vi "Create HTML.vi"(7 "FP Reference":refnum<class "Web Front Panel.lvclass">, 8 "error in (no error)":errorcluster, 10 "VI Identifier":string, 11 "Select In":refnum<class "Select.lvclass">) -> (0 "error out":errorcluster, 1 "js code for controls":string, 2 "js variables":string, 3 "Select Out":refnum<class "Select.lvclass">, 4 "script dependencies":string[](array[string]), 5 "HTML":string, 6 "js code for indicators":string)   [LabVIEW 2017, in "Front Panel Publisher.lvlib" / "Select.lvclass"]
uses:
  Select.lvclass
  Object_class/Object.lvclass
  Control_class/Control.lvclass
  Front Panel Publisher.lvlib
  Web Front Panel_class/Web Front Panel.lvclass
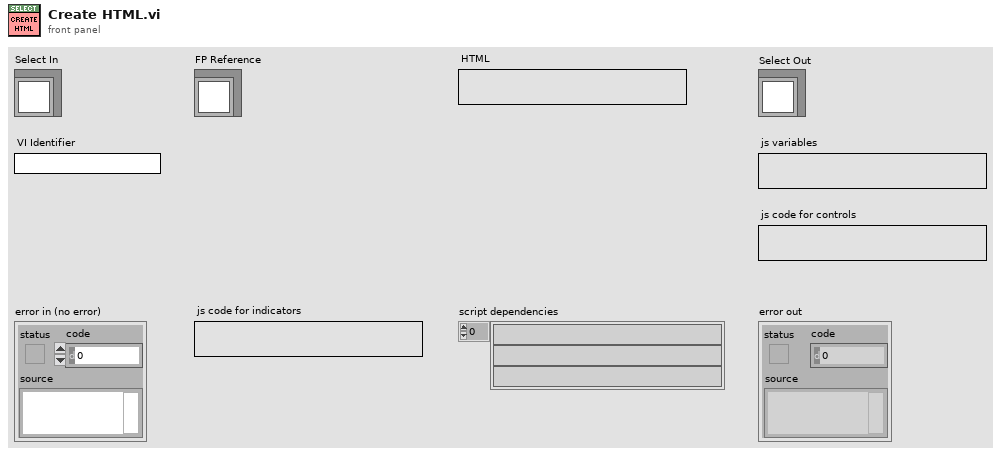
[diagram p1: front panel]
types:
  T1 = typedef "Front Panel Publisher.lvlib/Object.lvclass/Attributes.ctl" = cluster{"UID":i32, "Type":string, "Starting Location":T2, "Reference":refnum<vi>, "Cluster Component":bool, "Starting Rect Position":cluster{"Left":i16, "Top":i16}, "Owning Pane":refnum<vi>, "Master Total Rect Delta":T3}
  T2 = typedef "Front Panel Publisher.lvlib/Object.lvclass/Coordinates.ctl" = cluster{"Left":i32, "Top":i32, "Height":u32, "Width":u32}
  T3 = typedef "LVRectTypeDef.ctl" = cluster{"Left":i16, "Top":i16, "Right":i16, "Bottom":i16}
  T4 = typedef "Front Panel Publisher.lvlib/Control.lvclass/Attributes.ctl" = cluster{"Description":string, "Indicator":bool, "Default Value":variant, "Control Index":i32, "Label":refnum<class "Text.lvclass">, "Caption":refnum<class "Text.lvclass">, "Image b64":string, "No Control Index":bool, "Display Mode":T5}
  T5 = typedef "Front Panel Publisher.lvlib/Web Front Panel.lvclass/Enum - Control Display Mode.ctl" = enum16{"Value Only", "Value and Visibility", "Boolean Value Only", "Boolean Value and Visibility", "Control is Image", "Image and Visibility"}
  T6 = typedef "Front Panel Publisher.lvlib/Select.lvclass/Attributes.ctl" = cluster{"Ring Image Variable Name":string}
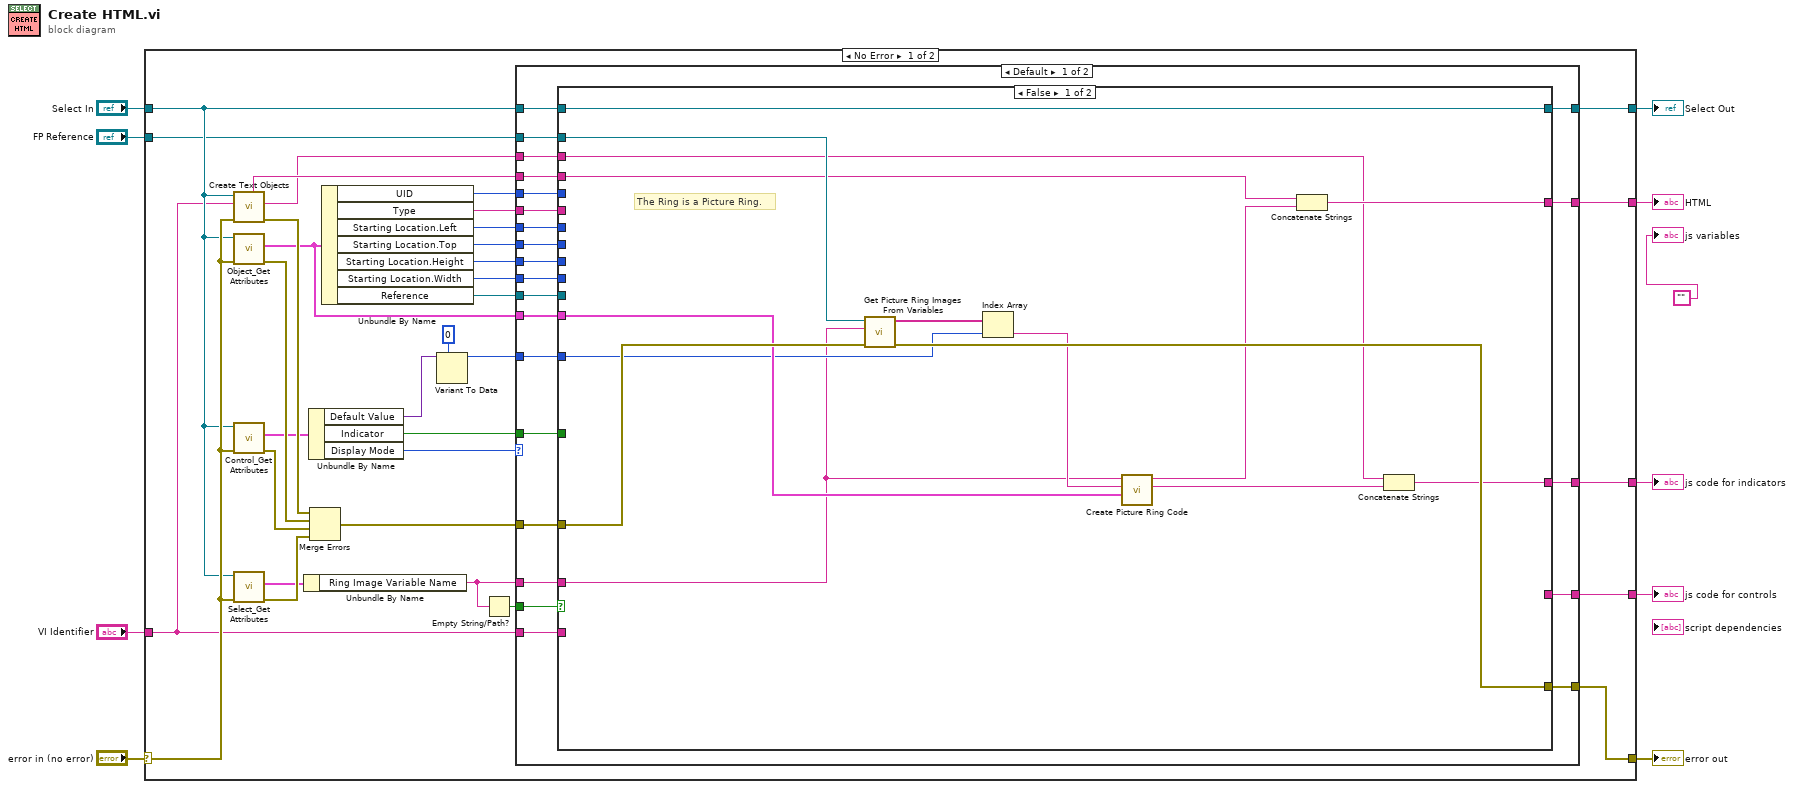
[diagram p0: block diagram]
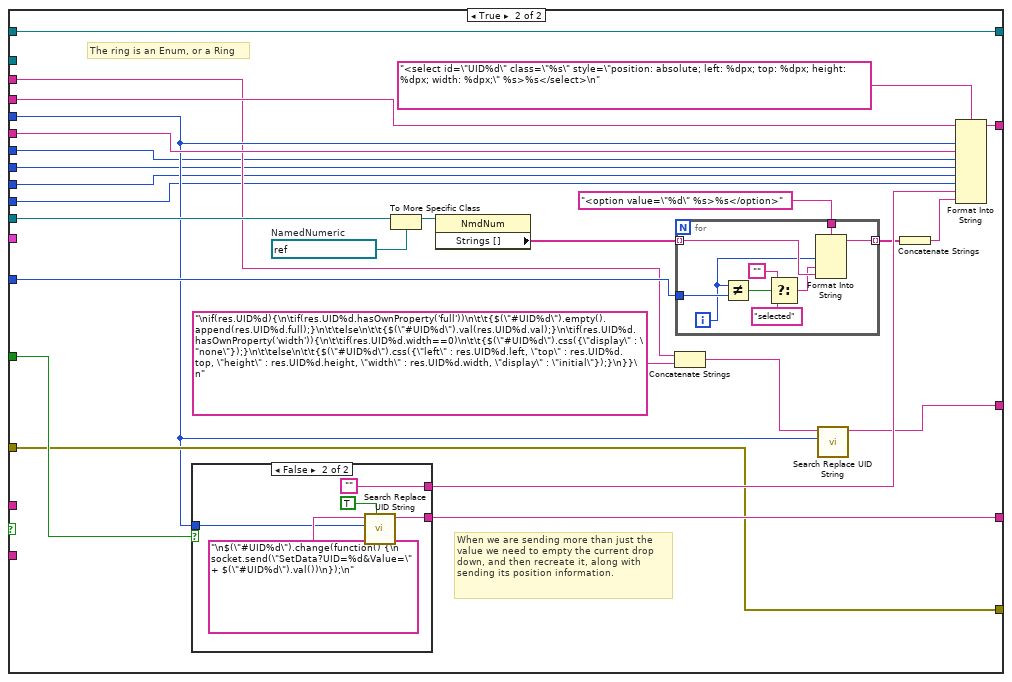
[diagram p2: hidden frame]
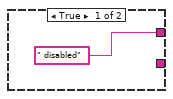
[diagram p3: hidden frame]
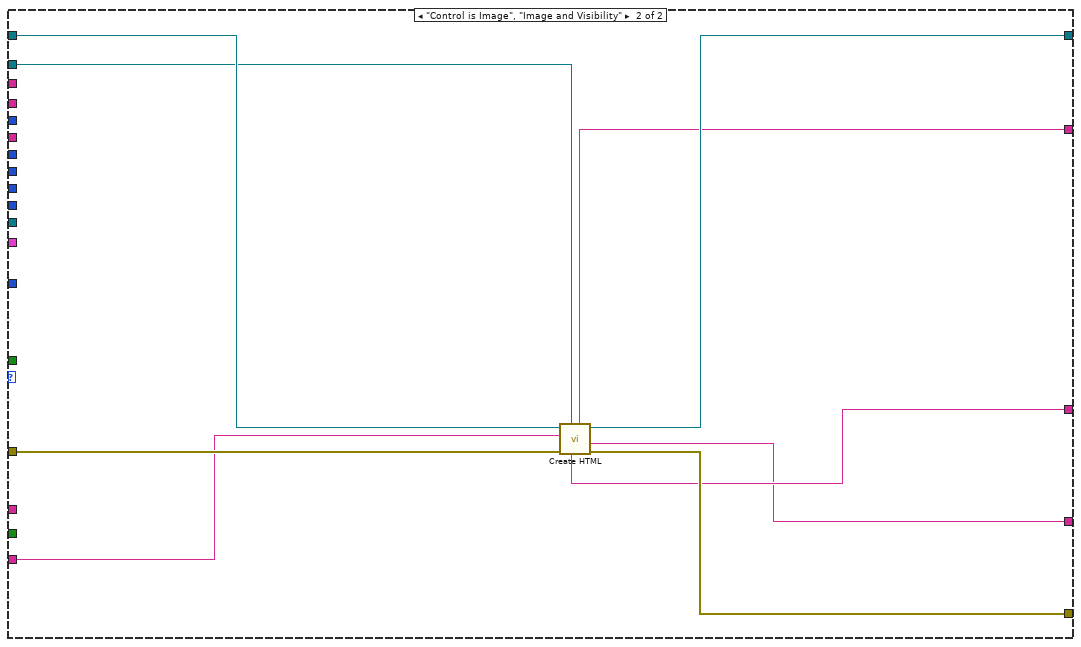
[diagram p4: hidden frame]
diagram:
  n1 = case shown="No Error" "error in (no error)" {
    selector: "error in (no error)" -> [w28 w133]
    tunnel: [w19 w133] -> w9
    tunnel: [w23 w132] -> w7
    tunnel: "Select In" -> [w24 w132]
    tunnel: [w38 _] -> w6
    tunnel: [w34 _] -> w5
    tunnel: [w35 _] -> w4
    tunnel: "VI Identifier" -> [w18 _]
    tunnel: "FP Reference" -> [w17 _]
    frame No Error {
      n2 = call-dynamic "Create Text Objects.vi"("error in (no error)"=w28, "VI Name"=w18, "Control In"=w24) -> ("error out"=w41:errorcluster, "JS Indicator"=w15:string, "HTML"=w33:string)  [unwired: 5 in, 1 out]
      n3 = call "Object_Get Attributes.vi"("error in (no error)"=w28, "Object In"=w24) -> ("error out"=w42:errorcluster, "Object Attributes"=w16:T1)  [unwired: 7 in, 1 out]
      n4 = call "Control_Get Attributes.vi"("error in (no error)"=w28, "Control In"=w24) -> ("error out"=w43:errorcluster, "Control Attributes"=w37:T4)  [unwired: 7 in, 1 out]
      n5 = call "Select_Get Attributes.vi"("error in (no error)"=w28, "Select In"=w24) -> ("error out"=w27:errorcluster, "Select Attributes"=w26:T6)  [unwired: 7 in, 1 out]
      n6 = Unbundle By Name(w26) -> ("Ring Image Variable Name"=w22:string)
      n7 = Unbundle By Name(w37) -> ("Default Value"=w31:variant, "Indicator"=w36:bool, "Display Mode"=w21:T5)
      n8 = Merge Errors(w41, w42, w43, w27) -> (w20:errorcluster)
      n9 = Unbundle By Name(w16) -> ("UID"=w40:i32, "Type"=w39:string, "Starting Location.Left"=w14:i32, "Starting Location.Top"=w13:i32, "Starting Location.Height"=w12:u32, "Starting Location.Width"=w11:u32, "Reference"=w32:refnum<vi>)
      n10 = Variant To Data(type=0, Variant=w31) -> (data=w29:i32)  [unwired: 1 in, 1 out]
      n11 = Empty String/Path?(string/path=w22) -> (empty?=w25:bool)
      n12 = case shown="Default" w21 {
        tunnel: w40 -> [w66 _]
        tunnel: w39 -> [w65 _]
        tunnel: [w64 w125] -> w38
        tunnel: w36 -> [w63 _]
        tunnel: [w62 w123] -> w35
        tunnel: [w61 w124] -> w34
        tunnel: w33 -> [w60 _]
        tunnel: w32 -> [w59 _]
        tunnel: w29 -> [w58 _]
        tunnel: w25 -> [w57 _]
        tunnel: w24 -> [w56 w129]
        tunnel: [w55 w126] -> w23
        tunnel: w22 -> [w54 _]
        tunnel: w20 -> [w53 w131]
        tunnel: [w52 w127] -> w19
        tunnel: w18 -> [w51 w130]
        tunnel: w17 -> [w50 w128]
        tunnel: w16 -> [w49 _]
        tunnel: w15 -> [w48 _]
        tunnel: w14 -> [w47 _]
        tunnel: w13 -> [w46 _]
        tunnel: w12 -> [w45 _]
        tunnel: w11 -> [w44 _]
        frame Default {
          n13 = case shown="False" w57 {
            tunnel: w66 -> [_ w89]
            tunnel: w65 -> [_ w106]
            tunnel: [w69 w105] -> w64
            tunnel: w63 -> [_ w104]
            tunnel: [_ w102] -> w62
            tunnel: [w70 w101] -> w61
            tunnel: w60 -> [w68 w100]
            tunnel: w59 -> [_ w99]
            tunnel: w58 -> [w73 w94]
            tunnel: w56 -> [w75 w91]
            tunnel: [w75 w91] -> w55
            tunnel: w54 -> [w71 _]
            tunnel: w53 -> [w81 w90]
            tunnel: [w80 w90] -> w52
            tunnel: w51 -> [_ _]
            tunnel: w50 -> [w77 _]
            tunnel: w49 -> [w76 _]
            tunnel: w48 -> [w67 w88]
            tunnel: w47 -> [_ w85]
            tunnel: w46 -> [_ w84]
            tunnel: w45 -> [_ w83]
            tunnel: w44 -> [_ w82]
            frame False {
              # "The Ring is a Picture Ring."
              n14 = call "Get Picture Ring Images From Variables.vi"("error in (no error)"=w81, "Ring Image Variable Name"=w71, "Web FP In"=w77) -> ("error out"=w80:errorcluster, "Images"=w74:string[])  [unwired: 7 in]
              n15 = Index Array(array=w74, index=w73) -> (element=w72:string)
              n16 = call "Create Picture Ring Code.vi"("Object Data"=w76, "Ring Image Default Image"=w72, "Ring Image Variable Name"=w71) -> ("JS Code For Indicators"=w78:string, "HTML"=w79:string)  [unwired: 7 in]
              n17 = Concatenate Strings(w68, w79) -> (w69:string)
              n18 = Concatenate Strings(w67, w78) -> (w70:string)
            }
            frame True {
              w97 = refnum<vi> refnum  # NamedNumeric
              # "The ring is an Enum, or a Ring"
              # "When we are sending more than just the value we need to empty the current drop down, and then recreate it, along with sending its position information."
              n19 = case shown="False" w104 {
                tunnel: [" disabled" ""] -> w103
                tunnel: w89 -> [_ w111]
                tunnel: [_ w110] -> w102
                frame True {
                }
                frame False {
                  n20 = call "Search Replace UID String.vi"("Replace All Numeric Inputs"=TRUE, "UID"=w111, "Input String"="\n$(\"#UID%d\").change(function() {\n  socket.send(\"SetData?UID=%d&Value=\" + $(\"#UID%d\").val())\n});\n") -> ("Output String"=w110:string)  [unwired: 8 in]
                }
              }
              n21 = To More Specific Class(target class=w97, reference=w99) -> (specific class reference=w98:refnum<vi>)  [unwired: 1 in, 1 out]
              n22 = property class="NmdNum"(reference=w98) -> ("Strings []"=w96:string[])  [unwired: 1 in, 2 out]
              n23 = Concatenate Strings(w88, "\nif(res.UID%d){\n\tif(res.UID%d.hasOwnProperty('full'))\n\t\t{$(\"#UID%d\").empty().append(res.UID%d.full);}\n\t\telse\n\t\t{$(\"#UID%d\").val(res.UID%d.val);}\n\tif(res.UID%d.hasOwnProperty('width')){\n\t\tif(res.UID%d.width==0)\n\t\t{$(\"#UID%d\").css({\"display\" : \"none\"});}\n\t\telse\n\t\t{$(\"#UID%d\").css({\"left\" : res.UID%d.left, \"top\" : res.UID%d.top, \"height\" : res.UID%d.height, \"width\" : res.UID%d.width, \"display\" : \"initial\"});}\n}}\n") -> (w87:string)
              n24 = for {
                tunnel: w96 -> [w121] mode=indexing
                tunnel: "<option value=\"%d\" %s>%s</option>" -> [w122]
                tunnel: w94 -> [w119]
                tunnel: [w117] -> w93 mode=indexing
                i -> [w116]
                n25 = Not Equal?(x=w116, y=w119) -> (x != y?=w120:bool)
                n26 = Select(t="", s=w120, f="selected") -> (s? t:f=w118:string)
                n27 = Format Into String(format string=w122, w116, w118, w121) -> (resulting string=w117:string)  [unwired: 2 in, 1 out]
              }
              n28 = call "Search Replace UID String.vi"("UID"=w89, "Input String"=w87) -> ("Output String"=w101:string)  [unwired: 9 in]
              n29 = Concatenate Strings(w93) -> (w92:string)
              n30 = Format Into String(format string="<select id=\"UID%d\" class=\"%s\" style=\"position: absolute; left: %dpx; top: %dpx; height: %dpx; width: %dpx;\" %s>%s</select>\n", initial string=w100, w89, w106, w85, w84, w83, w82, w103, w92) -> (resulting string=w105:string)  [unwired: 1 in, 1 out]
            }
          }
        }
        frame "Control is Image", "Image and Visibility" {
          n31 = call-parent "Create HTML.vi"("FP Reference"=w128, "error in (no error)"=w131, "VI Identifier"=w130, "Control In"=w129) -> ("error out"=w127:errorcluster, "js code for controls"=w123:string, "Control Out"=w126:refnum<class "Select.lvclass">, "HTML"=w125:string, "js code for indicators"=w124:string)  [unwired: 1 in, 2 out]
        }
      }
    }
    frame Error {
    }
  }
  "error out" <- w9
  "Select Out" <- w7
  "HTML" <- w6
  "js code for controls" <- w4
  "js code for indicators" <- w5
  "js variables" <- ""
